vi "CreateOutputTunnels.vi"(6 "error in":errorcluster, 9 "Loop in":refnum<class "Loop.lvclass">) -> (0 "error out":errorcluster, 3 "Loop out":refnum<class "Loop.lvclass">, 4 "createTunnels":string)   [LabVIEW 2014, in "Raspberry Pi Compatible Compiler for LabVIEW.lvlib" / "Loop.lvclass"]
uses:
  Loop.lvclass
  Python/Parsing/ClassTypeTD.ctl
  Python/Parsing/ListTypesTD.ctl
  LoopTunnel/LoopTunnel.lvclass/LoopTunnel.ctl
  Tunnel/Tunnel.lvclass/Tunnel.ctl
  LoopTunnel/LoopTunnel.lvclass
  Python/Parsing/Python Functions.lvlib
  Terminal/Terminal.lvclass
  Tunnel/Tunnel.lvclass
panel:
  in  "controlling":bool
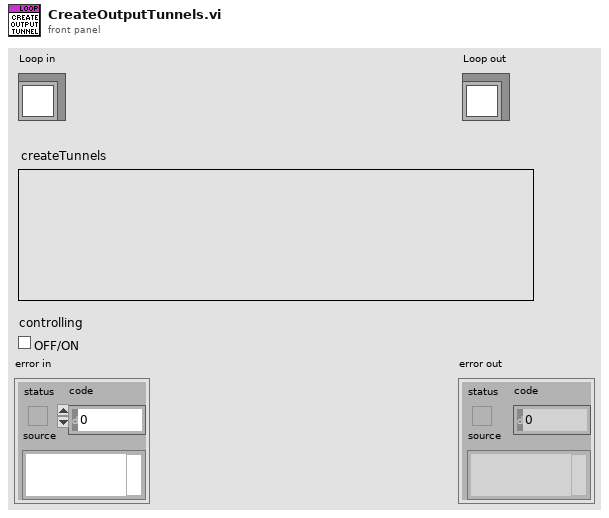
[diagram p1: front panel]
types:
  T1 = typedef "Raspberry Pi Compatible Compiler for LabVIEW.lvlib/Python Functions.lvlib/ListTypesTD.ctl" = enum16{"list", "tuple", "parameter list", "output list", "return values"}
  T2 = typedef "Raspberry Pi Compatible Compiler for LabVIEW.lvlib/Python Functions.lvlib/ClassTypeTD.ctl" = enum16{"class", "function"}
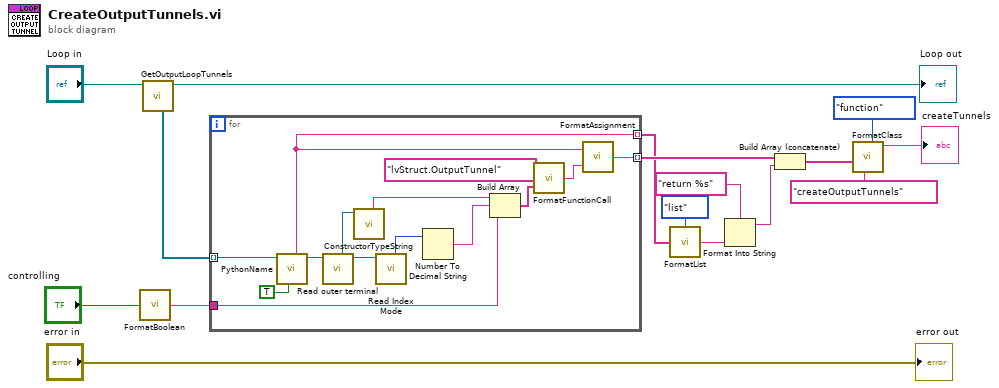
[diagram p0: block diagram]
diagram:
  n1 = call "FormatBoolean.vi"("value"="controlling") -> ("python object"=w7:string)
  n2 = call-dynamic "GetOutputLoopTunnels.vi"("Loop in"="Loop in") -> ("Loop out"=→"Loop out":refnum<class "Loop.lvclass">, "tunnels"=w11:refnum<class "LoopTunnel.lvclass">[])  [unwired: 6 in, 1 out]
  n3 = for {
    tunnel: w11 -> [w19] mode=indexing
    tunnel: [w27] -> w10 mode=indexing
    tunnel: w7 -> [w23]
    tunnel: [w17] -> w3 mode=indexing
    n4 = call-dynamic "PythonName.vi"("add self"=TRUE, "GObject in"=w19) -> ("GObject out"=w18:refnum<class "LoopTunnel.lvclass">, "name"=w17:string)  [unwired: 6 in, 2 out]
    n5 = call "Read outer terminal.vi"("Tunnel in"=w18) -> ("Tunnel out"=w29:refnum<class "LoopTunnel.lvclass">, "outer terminal"=w20:refnum<class "Terminal.lvclass">)  [unwired: 7 in]
    n6 = call "ConstructorTypeString.vi"("Terminal in"=w20) -> ("constructor string"=w25:string)  [unwired: 6 in, 2 out]
    n7 = call "Read Index Mode.vi"("LoopTunnel in"=w29) -> ("Index Mode"=w22:u32)  [unwired: 7 in, 1 out]
    n8 = Number To Decimal String(number=w22) -> (decimal integer string=w21:string)  [unwired: 1 in]
    n9 = Build Array(w25, w21, w23) -> (w24:string[])
    n10 = call "FormatFunctionCall.vi"("parameters"=w24, "function"="lvStruct.OutputTunnel" ("format string")) -> ("python object"=w26:string)
    n11 = call "FormatAssignment.vi"("value"=w26, "name"=w17) -> ("python assignment"=w27:string)
  }
  n12 = call "FormatList.vi"("values"=w3, "type"=ListTypesTD."list") -> ("python object"=w5:string)
  n13 = Format Into String(format string="return %s", w5) -> (resulting string=w1:string)  [unwired: 2 in, 1 out]
  n14 = Build Array (concatenate)(w10, w1) -> (w2:string[])
  n15 = call "FormatClass.vi"("type"=ClassTypeTD."function", "name"="createOutputTunnels", "body"=w2) -> ("python"=→"createTunnels":string)  [unwired: 8 in]
  "error out" <- "error in"
